vi "Merge Error.vi"(10 "Error":errorcluster, 11 "Set Error in":refnum<class "Actor.lvclass">) -> (3 "Set Error out":refnum<class "Actor.lvclass">)   [LabVIEW 2021, in "jettl.lvlib" / "Actor.lvclass"]
uses:
  Actor.lvclass
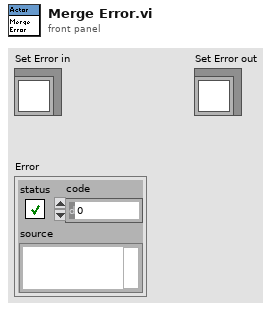
[diagram p1: front panel]
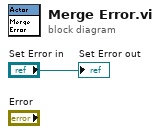
[diagram p0: block diagram]
diagram:
  "Set Error out" <- "Set Error in"
